vi "X Ray Expose On.vi"(8 "error in (no error)":errorcluster, 11 "nSensorIP":u32) -> (0 "error out":errorcluster, 3 "function return":i32)   [LabVIEW 2017, in "imgAcquisition.lvlib"]
doc: "DLLFunction int __stdcall ImageCapXRayExposeOn(unsigned int nSensorIP);"
uses:
  imgAcquisition.lvlib
  lib/ImageCaptureDLL.dll
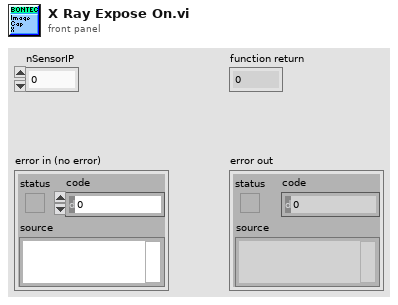
[diagram p1: front panel]
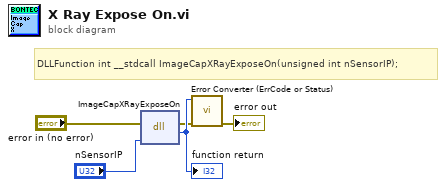
[diagram p0: block diagram]
diagram:
  # "DLLFunction int __stdcall ImageCapXRayExposeOn(unsigned int nSensorIP);"
  n1 = dll-call lib="F:/BonTechFlatPanelLVDriver/lib/ImageCaptureDLL.*" fn="ImageCapXRayExposeOn"(error in="error in (no error)", "nSensorIP"="nSensorIP") -> (error out=w2:errorcluster, w5:i32)  [unwired: 3 in, 1 out]
  "function return" <- w5
  n2 = call "Error Converter (ErrCode or Status).vi"("error in (no error)"=w2, "error code"=w5) -> ("error out"=→"error out":errorcluster)  [unwired: 9 in]
